vi "LevyLab Instrument.Configuration Window.vi"(8 "error in (no error)":errorcluster, 11 "Example Instrument in":refnum<class "Example.lvclass">) -> (0 "error out":errorcluster, 3 "Example Instrument out":refnum<class "Example.lvclass">)   [LabVIEW 2019, in "Example.lvclass"]
uses:
  Example.lvclass
  Example.lvclass/Example.ctl
panel:
  in  "Example Setting 3":string
  in  "Example Setting 2":dbl
  in  "Example Setting 1":dbl
  in  "Cancel":bool
  in  "OK":bool
  # "confirm or make changes:"
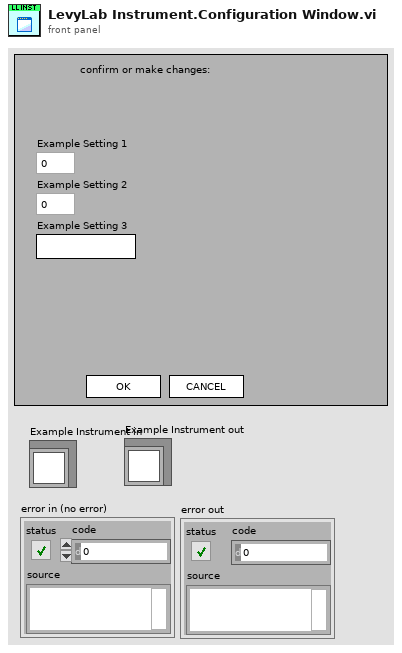
[diagram p1: front panel]
types:
  T1 = enum32{"Invalid", "Standard", "Closed", "Hidden", "Minimized", "Maximized"}
  T2 = enum32{"invalid app kind", "Development System", "Run Time System", "Student Edition", "Embedded LabVIEW", "Evaluation", "Custom"}
  T3 = typedef "Example.lvclass/LevyLab Instrument.Configuration--Cluster.ctl" = cluster{"Example Setting 1":dbl, "Example Setting 2":dbl, "Example Setting 3":string}
  T4 = cluster{"Core":cluster{"Current VI Reference":refnum<vi>, "Close Panel on Exit?":bool}, "Configuration":T3}
  T5 = cluster{"Current VI Reference":refnum<vi>, "Close Panel on Exit?":bool}
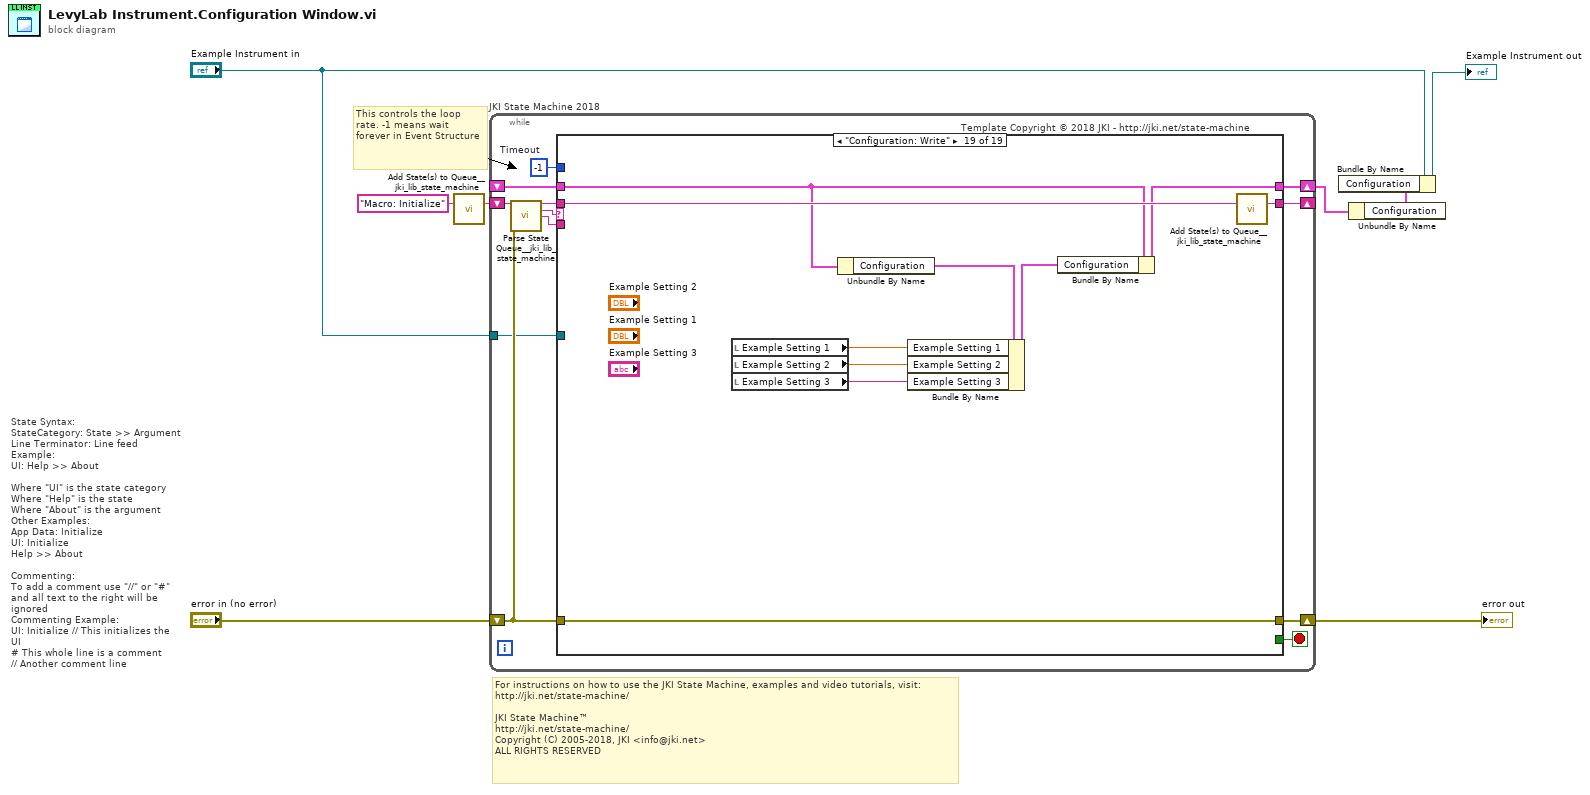
[diagram p0: block diagram]
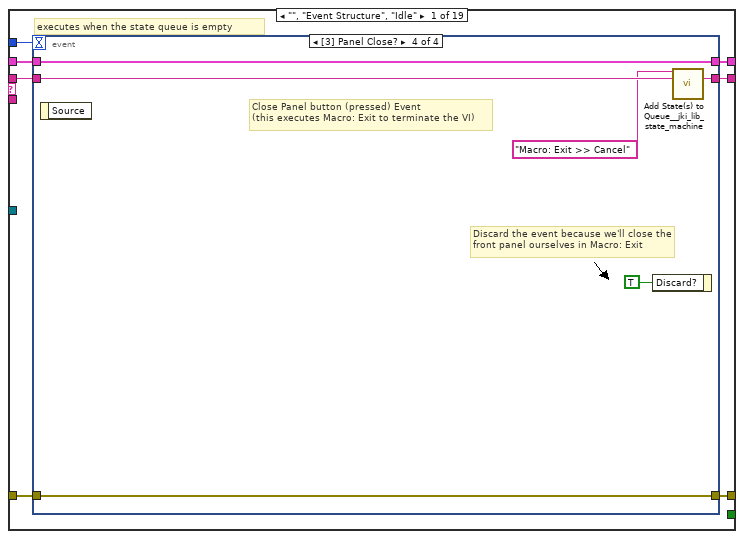
[diagram p2: hidden frame]
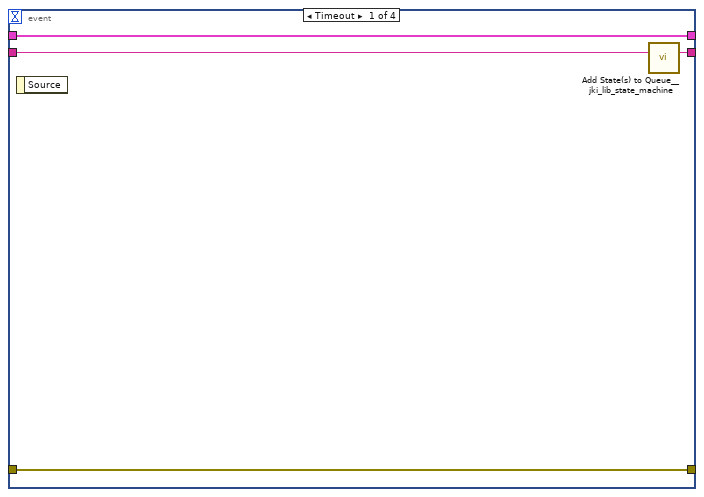
[diagram p3: hidden frame]
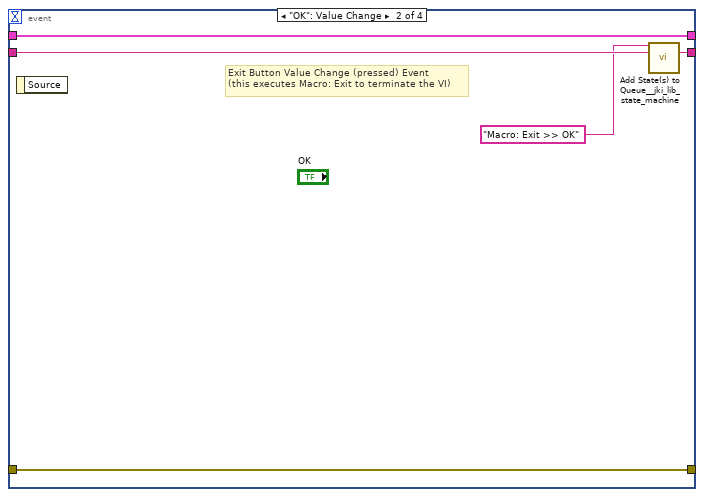
[diagram p4: hidden frame]
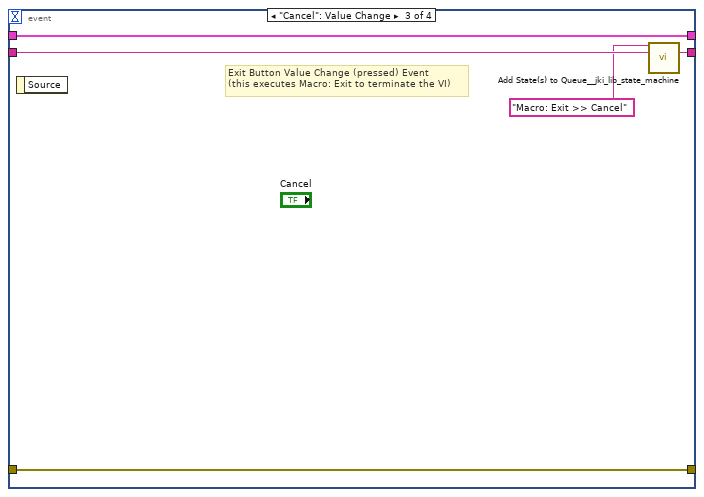
[diagram p5: hidden frame]
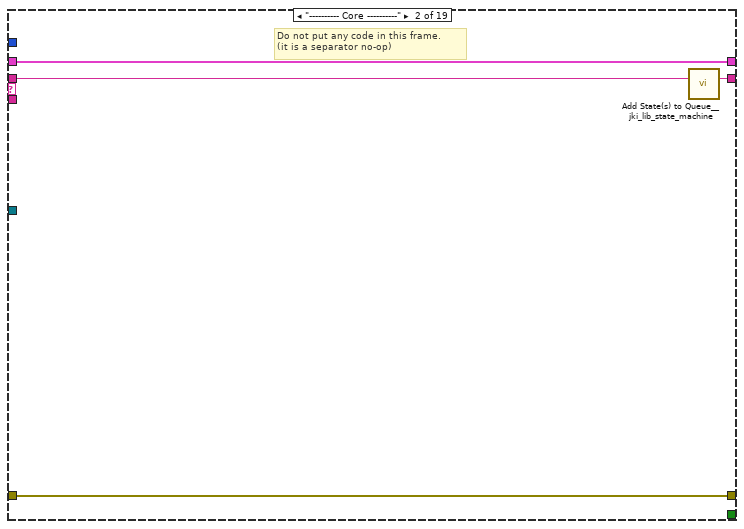
[diagram p6: hidden frame]
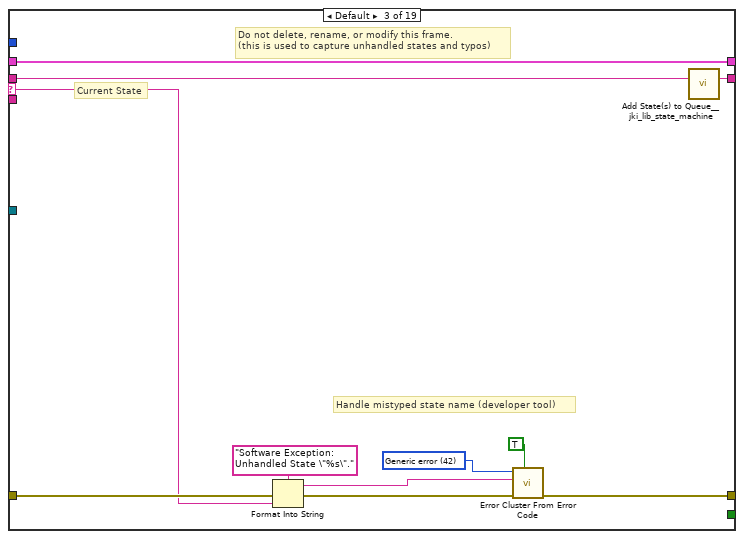
[diagram p7: hidden frame]
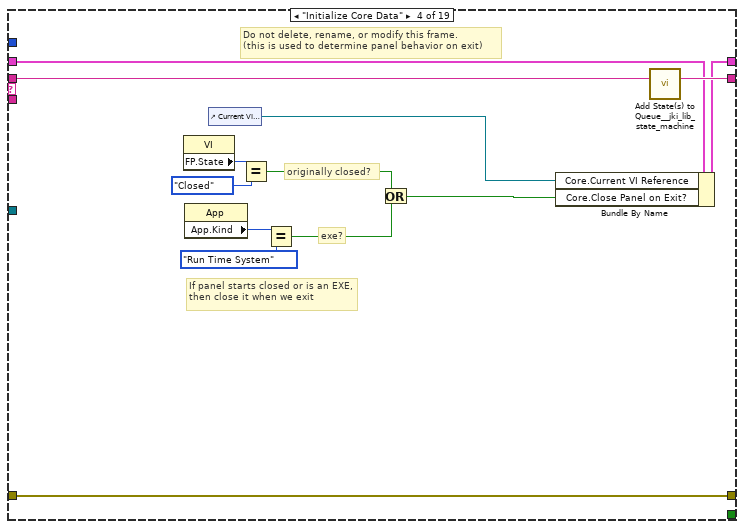
[diagram p8: hidden frame]
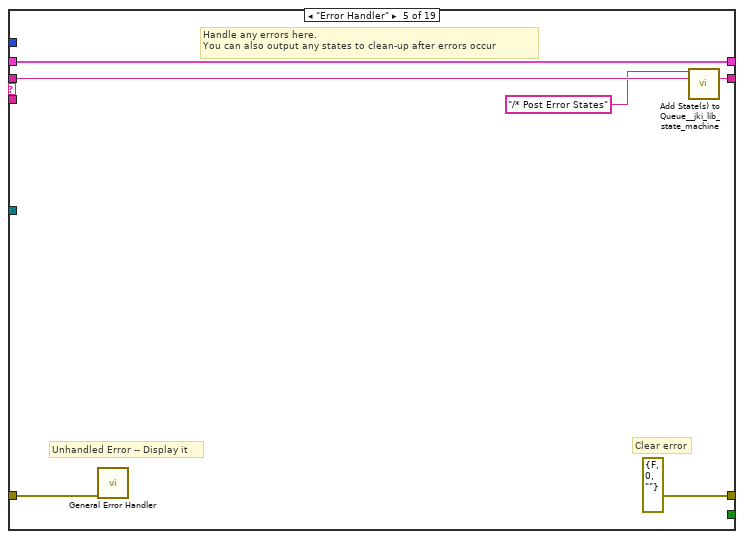
[diagram p9: hidden frame]
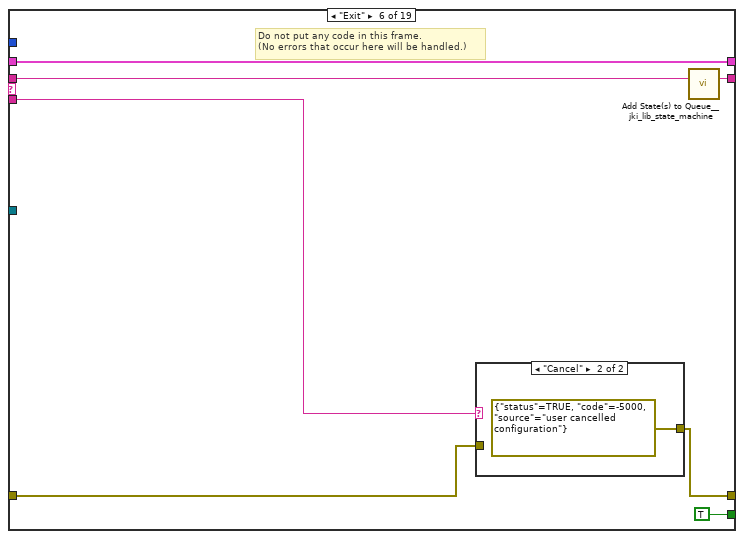
[diagram p10: hidden frame]
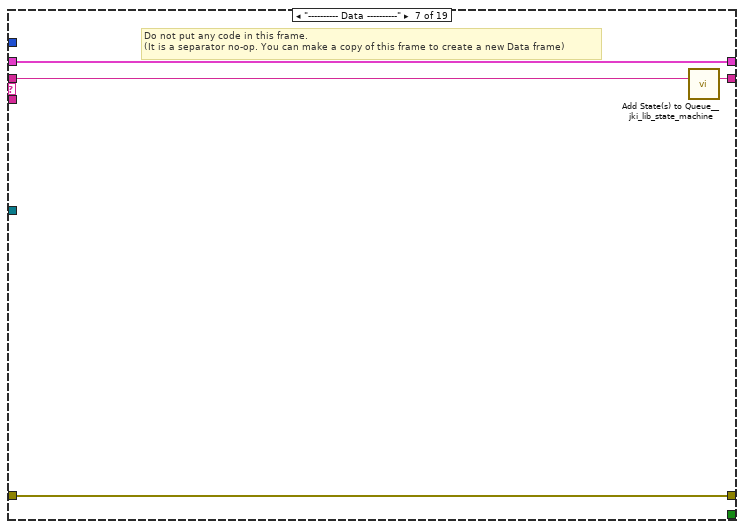
[diagram p12: hidden frame]
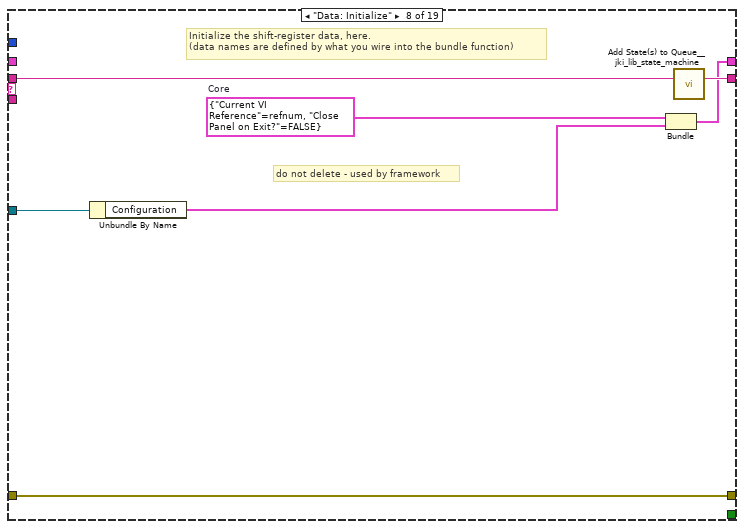
[diagram p13: hidden frame]
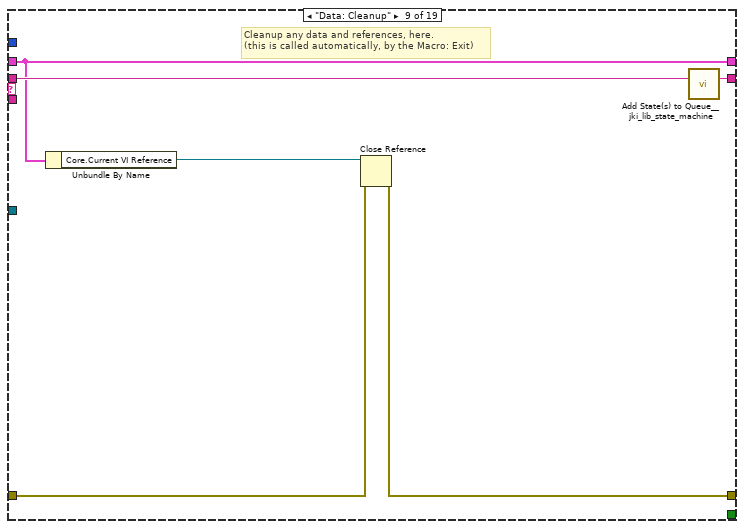
[diagram p14: hidden frame]
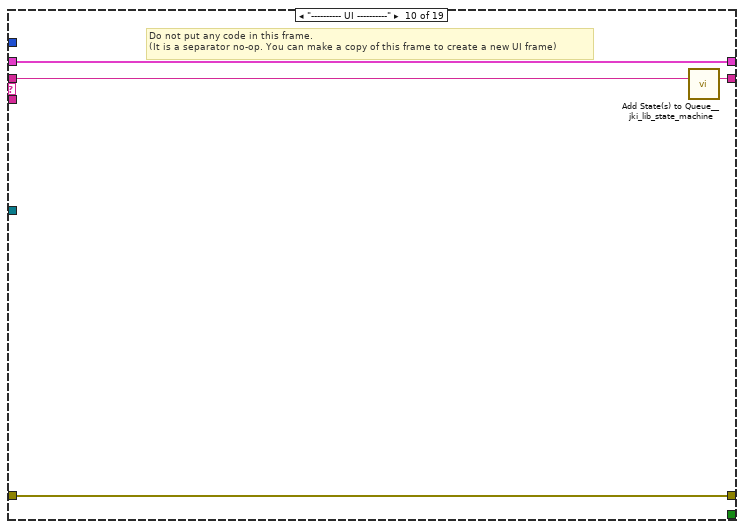
[diagram p15: hidden frame]
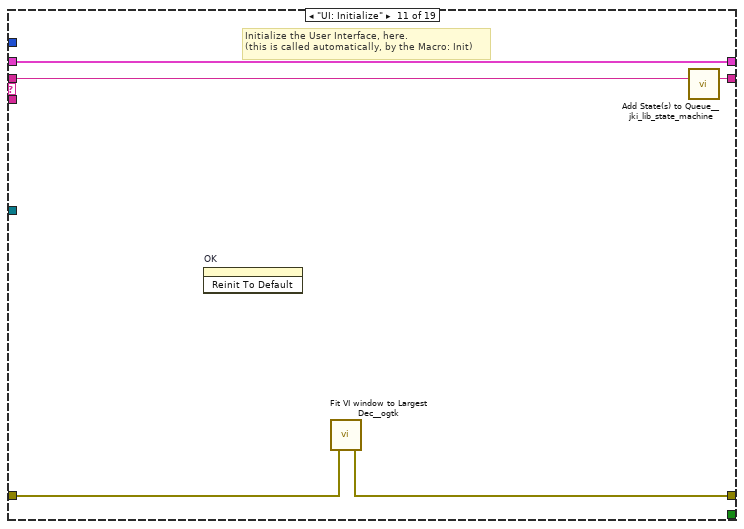
[diagram p16: hidden frame]
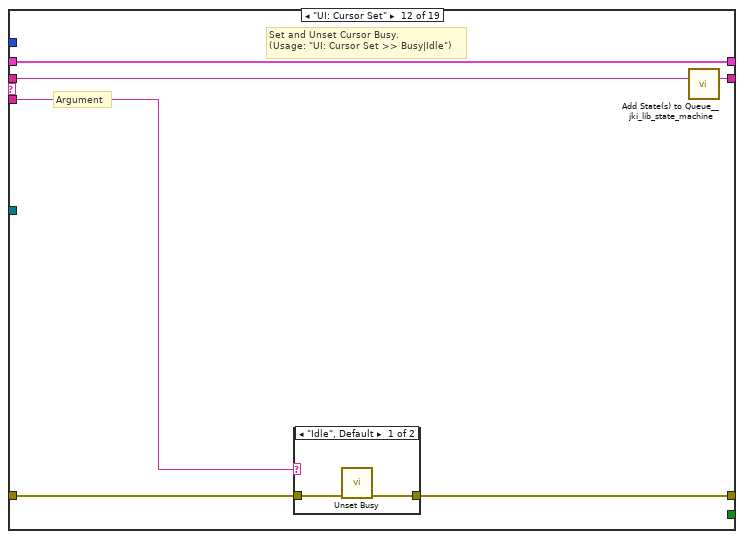
[diagram p17: hidden frame]
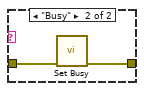
[diagram p18: hidden frame]
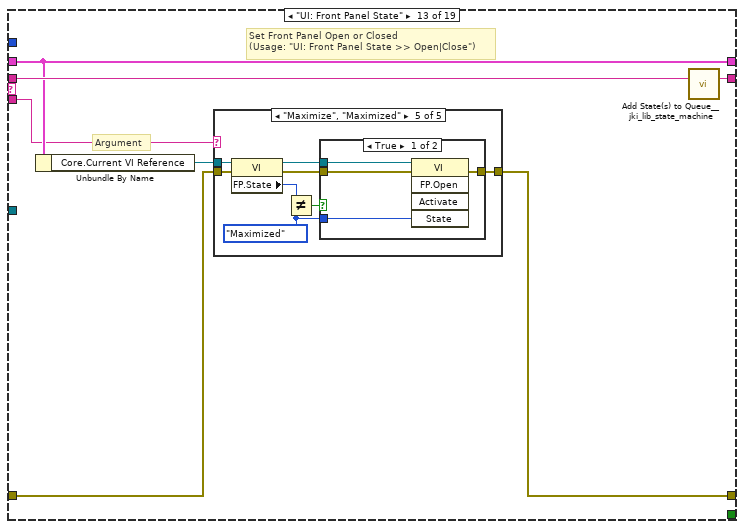
[diagram p19: hidden frame]
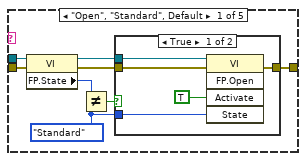
[diagram p20: hidden frame]
diagram:
  # "For instructions on how to use the JKI State Machine, examples and video tutorials, visit:\nhttp://jki.net/state-machine/\n\nJKI State Machine™\nhttp://jki.net/state-machine/\nCopyright (C) 2005-2018, JKI <info@jki.net>\nALL RIGHTS RESERVED"
  # "State Syntax:\nStateCategory: State >> Argument\nLine Terminator: Line feed\nExample:\nUI: Help >> About\n\nWhere \"UI\" is the state category\nWhere \"Help\" is the state\nWhere \"About\" is the argument\nOther Examples:\nApp Data: Initialize\nUI: Initialize\nHelp >> About\n\nCommenting:\nTo add a comment use \"//\" or \"#\" and all text to the right will be ignored\nCommenting Example:\nUI: Initialize // This initializes the UI\n# This whole line is a comment\n// Another comment line"
  # "This controls the loop rate. -1 means wait forever in Event Structure"
  n1 = call <vilib>:"Add State(s) to Queue__jki_lib_state_machine.vi"("State(s) in (\"\")"="Macro: Initialize") -> ("States Out"=w8:string)  [unwired: 14 in]
  n2 = while "JKI State Machine 2018" {
    shift-right: [w13] -> w2
    shift-left: _ -> [w12]
    shift-right: [w16] -> w6
    shift-left: "error in (no error)" -> [w10]
    shift-right: [w15] -> _
    shift-left: w8 -> [w17]
    tunnel: "Example Instrument in" -> [w9]
    stop <- w14 stop-if-true
    w11 = -1  # Timeout
    # "Template Copyright © 2018 JKI - http://jki.net/state-machine"
    n3 = call <vilib>:"Parse State Queue__jki_lib_state_machine.vi"("State Queue"=w17, "Error In (no error)"=w10) -> ("Remaining States"=w19:string, "Current State"=w20:string, "Arguments"=w18:string)  [unwired: 11 in]
    n4 = case shown="\"Configuration: Write\"" w20 {
      selector: w20 -> [_ _ w52 _ _ _ _ _ _ _ _ _ _ _ _ _ _ _ _]
      tunnel: w19 -> [w27 w51 w56 w75 w81 w88 w94 w101 w107 w111 w116 w122 w133 w202 w207 w222 w226 w234 w244]
      tunnel: w18 -> [_ _ _ _ _ w84 _ _ _ _ _ w117 w127 _ _ w211 _ _ _]
      tunnel: w12 -> [w25 w48 w54 w68 w78 w86 w91 _ w102 w108 w114 w120 w129 w199 w204 w219 w223 w228 w236]
      tunnel: [w24 w49 w58 w72 errorcluster {"status"=FALSE, "code"=0, "source"=""} ("error out") w82 w92 w97 w103 w109 w112 w118 w130 w200 w205 w220 w224 w232 w242] -> w16
      tunnel: w10 -> [w23 w49 w57 w72 w77 w83 w92 w97 w104 w109 w113 w119 w131 w200 w205 w220 w224 w232 w242]
      tunnel: [w26 w50 w55 w74 w80 w87 w93 w100 w106 w110 w115 w121 w132 w201 w206 w221 w225 w233 w243] -> w15
      tunnel: [_ _ _ _ _ TRUE _ _ _ _ _ _ _ _ _ _ _ _ _] -> w14
      tunnel: [w22 w48 w54 w73 w78 w86 w91 w99 w102 w108 w114 w120 w129 w199 w204 w219 w223 w228 w235] -> w13
      tunnel: w11 -> [w21 _ _ _ _ _ _ _ _ _ _ _ _ _ _ _ _ _ _]
      tunnel: w9 -> [_ _ _ _ _ _ _ w96 _ _ _ _ _ _ _ _ _ _ _]
      frame "", "Event Structure", "Idle" {
        # "executes when the state queue is empty"
        n5 = event shown="[3] Panel Close?" {
          selector: _ -> [_ _ _ _]
          dyn-events: _ -> [_ _ _ _]
          timeout: w21 -> [_ _ _ _]
          tunnel: w27 -> [w31 w36 w41 w47]
          tunnel: [w30 w35 w40 w46] -> w26
          tunnel: w25 -> [w28 w33 w38 w44]
          tunnel: [w29 w34 w39 w45] -> w24
          tunnel: w23 -> [w29 w34 w39 w45]
          tunnel: [w28 w33 w38 w44] -> w22
          event Timeout {
            n6 = event-data() -> ()  [unwired: 1 in, 1 out]
            n7 = call <vilib>:"Add State(s) to Queue__jki_lib_state_machine.vi"("State(s) in (\"\")"=w31) -> ("States Out"=w30:string)  [unwired: 14 in]
          }
          event "OK": Value Change {
            # "Exit Button Value Change (pressed) Event\n(this executes Macro: Exit to terminate the VI)"
            n8 = event-data() -> ()  [unwired: 1 in, 1 out]
            n9 = call <vilib>:"Add State(s) to Queue__jki_lib_state_machine.vi"("State(s) in Front (\"\")"="Macro: Exit >> OK", "State(s) in (\"\")"=w36) -> ("States Out"=w35:string)  [unwired: 13 in]
          }
          event "Cancel": Value Change {
            # "Exit Button Value Change (pressed) Event\n(this executes Macro: Exit to terminate the VI)"
            n10 = event-data() -> ()  [unwired: 1 in, 1 out]
            n11 = call <vilib>:"Add State(s) to Queue__jki_lib_state_machine.vi"("State(s) in Front (\"\")"="Macro: Exit >> Cancel", "State(s) in (\"\")"=w41) -> ("States Out"=w40:string)  [unwired: 13 in]
          }
          event Panel Close? {
            # "Discard the event because we'll close the front panel ourselves in Macro: Exit"
            # "Close Panel button (pressed) Event\n(this executes Macro: Exit to terminate the VI)"
            n12 = event-data() -> ()  [unwired: 1 in, 1 out]
            n13 = event-data("Discard?"=TRUE) -> ()  [unwired: 1 in, 1 out]
            n14 = call <vilib>:"Add State(s) to Queue__jki_lib_state_machine.vi"("State(s) in Front (\"\")"="Macro: Exit >> Cancel", "State(s) in (\"\")"=w47) -> ("States Out"=w46:string)  [unwired: 13 in]
          }
        }
      }
      frame "---------- Core ----------" {
        # "Do not put any code in this frame.\n(it is a separator no-op)"
        n15 = call <vilib>:"Add State(s) to Queue__jki_lib_state_machine.vi"("State(s) in (\"\")"=w51) -> ("States Out"=w50:string)  [unwired: 14 in]
      }
      frame Default {
        w61 = 42 items=["No error", "Argument error", "Memory is full", "Out of zone", "End of file", "File already open", "Generic file I/O error", "File not found", "File permission error", "Disk is full", "Duplicate path", "Too many files open", "System feature not enabled", "Resource file not found", "Cannot add resource", "Resource not found", "Image not found", "Image memory error", "Pen does not exist", "Config type invalid", "Config token not found", "Config parse error", "Config memory error", "Bad external code format", "Bad external code offset", "External code not present", "Null window", "Destroy window error", "Null menu", "Print aborted", "Bad print record", "Print driver error", "Windows error during printing", "Memory error during printing", "Print dialog error", "Generic print error", "Invalid device refnum", "Device not found", "Device parameter error", "Device unit error", "Cannot open device", "Device call aborted", "Generic error", "Cancelled by user", "Object ID too low", "Object ID too high", "Object not in heap", "Unknown heap", "Unknown object (invalid DefProc)", "Unknown object (DefProc not in table)", "Message out of range", "Invalid (null) method", "Unknown message", "Manager call not supported", "Bad address", "Network operation in progress", "Network operation timed out", "Connection is busy", "Network attribute not supported", "Network error", "Address in use", "System out of memory", "Connection aborted", "Connection refused", "Not connected", "Already connected", "Connection closed", "Initialization error (interapplication manager)", "Bad occurrence", "Wait on unbound occurrence handler", "Occurrence queue overflow", "Datalog type conflict", "Unused", "Unrecognized type (interapplication manager)", "Memory corrupt", "Failed to make temporary DLL", "Old CIN version", "Drag socket not found", "Failed to load drop-object", "Failed to register OLE object", "Failed to release OLE object", "Format specifier type mismatch", "Unknown format specifier", "Too few format specifiers", "Too many format specifiers", "Scan failed", "Newer CIN version", "Error converting to variant", "Runtime menu error", "Password tampered", "Variant attribute not found", "Incompatible variant data type", "Event data is not available", "Event Store is not present", "Occurrence is not found", "Event Queue is not created", "Event info is not available", "Refnum passed is NULL", "Error retrieving Class GUID", "Error retrieving CoClass GUID", "Error retrieving TypeLib GUID.", "Bad built application magic bytes.", "Specific driver is different from the specific driver associated with the Logical Name.", "There is no session opened to the class driver.", "Max Error", "MAX - Error with config objects", "MAX - Error loading configuration", "MAX - Group not supported"]
        # "Current State"
        # "Do not delete, rename, or modify this frame.\n(this is used to capture unhandled states and typos)"
        # "Handle mistyped state name (developer tool)"
        n16 = Format Into String(format string="Software Exception: Unhandled State \"%s\"." ("message"), error in=w57, w52) -> (resulting string=w60:string, error out=w59:errorcluster)  [unwired: 1 in]
        n17 = call <vilib>:"Error Cluster From Error Code.vi"("show call chain? (False)"=TRUE, "error in (no error)"=w59, "error message (\"\")"=w60, "error code (0)"=w61) -> ("error out"=w58:errorcluster)  [unwired: 5 in]
        n18 = call <vilib>:"Add State(s) to Queue__jki_lib_state_machine.vi"("State(s) in (\"\")"=w56) -> ("States Out"=w55:string)  [unwired: 14 in]
      }
      frame "Initialize Core Data" {
        # "Do not delete, rename, or modify this frame.\n(this is used to determine panel behavior on exit)"
        # "originally closed?"
        # "exe?"
        # "If panel starts closed or is an EXE, then close it when we exit"
        n19 = property class="VI"() -> ("FP.State"=w65:T1)  [unwired: 2 in, 2 out]
        n20 = property class="App"() -> ("App.Kind"=w71:T2)  [unwired: 2 in, 2 out]
        n21 = control-ref of="Current VI Reference"() -> (w66:refnum<vi>)
        n22 = Equal?(x=w65, y=T1."Closed" ("Front Panel Window:State")) -> (x = y?=w63:bool)
        n23 = Equal?(x=w71, y=T2."Run Time System" ("Application:Kind")) -> (x = y?=w69:bool)
        n24 = Or(x=w63, y=w69) -> (x .or. y?=w67:bool)
        n25 = Bundle By Name(cluster=w68, "Core.Current VI Reference"=w66, "Core.Close Panel on Exit?"=w67) -> (w73:T4)
        n26 = call <vilib>:"Add State(s) to Queue__jki_lib_state_machine.vi"("State(s) in (\"\")"=w75) -> ("States Out"=w74:string)  [unwired: 14 in]
      }
      frame "Error Handler" {
        # "Unhandled Error -- Display it"
        # "Handle any errors here.\nYou can also output any states to clean-up after errors occur"
        # "Clear error"
        n27 = call <vilib>:"General Error Handler.vi"("error in (no error)"=w77) -> ()  [unwired: 10 in, 5 out]
        n28 = call <vilib>:"Add State(s) to Queue__jki_lib_state_machine.vi"("State(s) in Front (\"\")"="/* Post Error States", "State(s) in (\"\")"=w81) -> ("States Out"=w80:string)  [unwired: 13 in]
      }
      frame "Exit" {
        # "Do not put any code in this frame.\n(No errors that occur here will be handled.)"
        n29 = case shown="\"Cancel\"" w84 {
          tunnel: w83 -> [w89 _]
          tunnel: [w89 errorcluster {"status"=TRUE, "code"=-5000, "source"="user cancelled configuration"} ("error in (no error)")] -> w82
          frame "OK", Default {
          }
          frame "Cancel" {
          }
        }
        n30 = call <vilib>:"Add State(s) to Queue__jki_lib_state_machine.vi"("State(s) in (\"\")"=w88) -> ("States Out"=w87:string)  [unwired: 14 in]
      }
      frame "---------- Data ----------" {
        # "Do not put any code in this frame.\n(It is a separator no-op. You can make a copy of this frame to create a new Data frame)"
        n31 = call <vilib>:"Add State(s) to Queue__jki_lib_state_machine.vi"("State(s) in (\"\")"=w94) -> ("States Out"=w93:string)  [unwired: 14 in]
      }
      frame "Data: Initialize" {
        w98 = T5 {"Current VI Reference"=refnum, "Close Panel on Exit?"=FALSE}  # Core
        # "do not delete - used by framework"
        # "Initialize the shift-register data, here.\n(data names are defined by what you wire into the bundle function)"
        n32 = Unbundle By Name(w96) -> ("Configuration"=w95:T3)
        n33 = Bundle("Core"=w98, "Configuration"=w95) -> (w99:T4)  [unwired: 1 in]
        n34 = call <vilib>:"Add State(s) to Queue__jki_lib_state_machine.vi"("State(s) in (\"\")"=w101) -> ("States Out"=w100:string)  [unwired: 14 in]
      }
      frame "Data: Cleanup" {
        # "Cleanup any data and references, here.\n(this is called automatically, by the Macro: Exit)"
        n35 = Unbundle By Name(w102) -> ("Core.Current VI Reference"=w105:refnum<vi>)
        n36 = Close Reference(reference=w105, error in (no error)=w104) -> (error out=w103:errorcluster)
        n37 = call <vilib>:"Add State(s) to Queue__jki_lib_state_machine.vi"("State(s) in (\"\")"=w107) -> ("States Out"=w106:string)  [unwired: 14 in]
      }
      frame "---------- UI ----------" {
        # "Do not put any code in this frame.\n(It is a separator no-op. You can make a copy of this frame to create a new UI frame)"
        n38 = call <vilib>:"Add State(s) to Queue__jki_lib_state_machine.vi"("State(s) in (\"\")"=w111) -> ("States Out"=w110:string)  [unwired: 14 in]
      }
      frame "UI: Initialize" {
        # "Initialize the User Interface, here.\n(this is called automatically, by the Macro: Init)"
        n39 = invoke on="OK" class="Bool" method="Reinit To Default"() -> ()  [unwired: 3 in, 3 out]
        n40 = call <userlib>:"Fit VI window to Largest Dec__ogtk.vi"("error in (no error)"=w113) -> ("error out"=w112:errorcluster)  [unwired: 5 in, 1 out]
        n41 = call <vilib>:"Add State(s) to Queue__jki_lib_state_machine.vi"("State(s) in (\"\")"=w116) -> ("States Out"=w115:string)  [unwired: 14 in]
      }
      frame "UI: Cursor Set" {
        # "Argument"
        # "Set and Unset Cursor Busy.\n(Usage: \"UI: Cursor Set >> Busy|Idle\")"
        n42 = case shown="\"Idle\", Default" w117 {
          tunnel: w119 -> [w124 w126]
          tunnel: [w123 w125] -> w118
          frame "Idle", Default {
            n43 = call <vilib>:"Unset Busy.vi"("error in (no error)"=w124) -> ("error out"=w123:errorcluster)  [unwired: 10 in]
          }
          frame "Busy" {
            n44 = call <vilib>:"Set Busy.vi"("error in (no error)"=w126) -> ("error out"=w125:errorcluster)  [unwired: 9 in, 1 out]
          }
        }
        n45 = call <vilib>:"Add State(s) to Queue__jki_lib_state_machine.vi"("State(s) in (\"\")"=w122) -> ("States Out"=w121:string)  [unwired: 14 in]
      }
      frame "UI: Front Panel State" {
        # "Argument"
        # "Set Front Panel Open or Closed\n(Usage: \"UI: Front Panel State >> Open|Close\")"
        n46 = Unbundle By Name(w129) -> ("Core.Current VI Reference"=w128:refnum<vi>)
        n47 = case shown="\"Maximize\", \"Maximized\"" w127 {
          tunnel: w131 -> [w139 w154 w165 w178 w191]
          tunnel: [w141 w155 w167 w180 w193] -> w130
          tunnel: w128 -> [w140 w152 w166 w179 w192]
          frame "Open", "Standard", Default {
            w134 = T1."Standard" ("State")
            n48 = property class="VI"(reference=w140, error in=w139) -> (reference out=w137:refnum<vi>, error out=w138:errorcluster, "FP.State"=w136:T1)
            n49 = Not Equal?(x=w136, y=w134) -> (x != y?=w135:bool)
            n50 = case shown="True" w135 {
              tunnel: [w145 w147] -> w141
              tunnel: w138 -> [w144 w147]
              tunnel: w137 -> [w143 _]
              tunnel: w134 -> [w142 _]
              frame True {
                n51 = invoke class="VI" method="FP.Open"(reference=w143, error in=w144, "Activate"=TRUE, "State"=w142) -> (error out=w145:errorcluster)  [unwired: 1 in, 4 out]
              }
              frame False {
              }
            }
          }
          frame "Close", "Closed" {
            n52 = property class="VI"(reference=w152, error in=w154) -> (reference out=w151:refnum<vi>, error out=w153:errorcluster, "FP.State"=w149:T1)
            n53 = Not Equal?(x=w149, y=T1."Closed" ("Front Panel Window:State")) -> (x != y?=w148:bool)
            n54 = case shown="True" w148 {
              tunnel: [w156 w159] -> w155
              tunnel: w153 -> [w156 w158]
              tunnel: w151 -> [_ w157]
              frame False {
              }
              frame True {
                n55 = invoke class="VI" method="FP.Close"(reference=w157, error in=w158) -> (error out=w159:errorcluster)  [unwired: 1 in, 2 out]
              }
            }
          }
          frame "Hidden", "Hide" {
            w160 = T1."Hidden" ("State")
            n56 = property class="VI"(reference=w166, error in=w165) -> (reference out=w163:refnum<vi>, error out=w164:errorcluster, "FP.State"=w162:T1)
            n57 = Not Equal?(x=w162, y=w160) -> (x != y?=w161:bool)
            n58 = case shown="True" w161 {
              tunnel: [w171 w172] -> w167
              tunnel: w164 -> [w170 w172]
              tunnel: w163 -> [w169 _]
              tunnel: w160 -> [w168 _]
              frame True {
                n59 = invoke class="VI" method="FP.Open"(reference=w169, error in=w170, "State"=w168) -> (error out=w171:errorcluster)  [unwired: 2 in, 4 out]
              }
              frame False {
              }
            }
          }
          frame "Minimize", "Minimized" {
            w173 = T1."Minimized" ("State")
            n60 = property class="VI"(reference=w179, error in=w178) -> (reference out=w176:refnum<vi>, error out=w177:errorcluster, "FP.State"=w175:T1)
            n61 = Not Equal?(x=w175, y=w173) -> (x != y?=w174:bool)
            n62 = case shown="True" w174 {
              tunnel: [w184 w185] -> w180
              tunnel: w177 -> [w183 w185]
              tunnel: w176 -> [w182 _]
              tunnel: w173 -> [w181 _]
              frame True {
                n63 = invoke class="VI" method="FP.Open"(reference=w182, error in=w183, "State"=w181) -> (error out=w184:errorcluster)  [unwired: 2 in, 4 out]
              }
              frame False {
              }
            }
          }
          frame "Maximize", "Maximized" {
            w186 = T1."Maximized" ("State")
            n64 = property class="VI"(reference=w192, error in=w191) -> (reference out=w189:refnum<vi>, error out=w190:errorcluster, "FP.State"=w188:T1)
            n65 = Not Equal?(x=w188, y=w186) -> (x != y?=w187:bool)
            n66 = case shown="True" w187 {
              tunnel: [w197 w198] -> w193
              tunnel: w190 -> [w196 w198]
              tunnel: w189 -> [w195 _]
              tunnel: w186 -> [w194 _]
              frame True {
                n67 = invoke class="VI" method="FP.Open"(reference=w195, error in=w196, "State"=w194) -> (error out=w197:errorcluster)  [unwired: 2 in, 4 out]
              }
              frame False {
              }
            }
          }
        }
        n68 = call <vilib>:"Add State(s) to Queue__jki_lib_state_machine.vi"("State(s) in (\"\")"=w133) -> ("States Out"=w132:string)  [unwired: 14 in]
      }
      frame "---------- Macro ----------" {
        # "Do not put any code in this frame.\n(It is a separator no-op. You can make a copy of this frame to create a new Macro frame)"
        n69 = call <vilib>:"Add State(s) to Queue__jki_lib_state_machine.vi"("State(s) in (\"\")"=w202) -> ("States Out"=w201:string)  [unwired: 14 in]
      }
      frame "Macro: Initialize" {
        w203 = "Data: Initialize\nInitialize Core Data\nUI: Initialize\nUI: Front Panel State >> Open\nConfiguration: Read"  # Data: Initialize Initialize Core Data UI: Initialize UI: Front Panel State >> Open Configuration: Read
        # "Initialization Macro\n(This is called once, when the VI starts)"
        n70 = call <vilib>:"Add State(s) to Queue__jki_lib_state_machine.vi"("State(s) in Front (\"\")"=w203, "State(s) in (\"\")"=w207) -> ("States Out"=w206:string)  [unwired: 13 in]
      }
      frame "Macro: Exit" {
        # "Exit Macro\n(This is called once, when the VI exits)"
        n71 = Unbundle By Name(w219) -> ("Core.Close Panel on Exit?"=w218:bool)
        n72 = call <vilib>:"Build State String with Arguments__JKI_lib_State_Machine.vi"("Arguments (\"\")"=w211, "State"="Exit") -> ("State with Arguments"=w209:string)  [unwired: 4 in]
        n73 = Select(t="UI: Front Panel State >> Close", s=w218, f="") -> (s? t:f=w215:string)
        n74 = call <vilib>:"Add State(s) to Queue__jki_lib_state_machine.vi"("State(s) in Front (\"\")"="Data: Cleanup", "State(s) at Back (\"\")"=w209) -> ("States Out"=w208:string)  [unwired: 13 in]
        n75 = call <vilib>:"Add State(s) to Queue__jki_lib_state_machine.vi"("State(s) in Front (\"\")"="Configuration: Write", "State(s) in (\"\")"=w215, "State(s) at Back (\"\")"=w208) -> ("States Out"=w214:string)  [unwired: 12 in]
        n76 = call <vilib>:"Add State(s) to Queue__jki_lib_state_machine.vi"("State(s) in Front (\"\")"=w214, "State(s) in (\"\")"=w222) -> ("States Out"=w221:string)  [unwired: 13 in]
      }
      frame "---------- Configuration ----------" {
        # "Template Separator\n(You can make a copy of, or modify, this frame)"
        n77 = call <vilib>:"Add State(s) to Queue__jki_lib_state_machine.vi"("State(s) in (\"\")"=w226) -> ("States Out"=w225:string)  [unwired: 14 in]
      }
      frame "Configuration: Read" {
        # "Your code here.\n(You can make a copy of, or modify, this frame)"
        n78 = Unbundle By Name(w228) -> ("Configuration"=w227:T3)
        n79 = Unbundle By Name(w227) -> ("Example Setting 1"=w231:dbl, "Example Setting 2"=w230:dbl, "Example Setting 3"=w229:string)
        n80 = local write "Example Setting 2"(w230) -> ()
        n81 = local write "Example Setting 1"(w231) -> ()
        n82 = local write "Example Setting 3"(w229) -> ()
        n83 = call <vilib>:"Add State(s) to Queue__jki_lib_state_machine.vi"("State(s) in (\"\")"=w234) -> ("States Out"=w233:string)  [unwired: 14 in]
      }
      frame "Configuration: Write" {
        n84 = local read "Example Setting 1"() -> (w241:dbl)
        n85 = local read "Example Setting 2"() -> (w238:dbl)
        n86 = local read "Example Setting 3"() -> (w239:string)
        n87 = Unbundle By Name(w236) -> ("Configuration"=w240:T3)
        n88 = Bundle By Name(cluster=w240, "Example Setting 1"=w241, "Example Setting 2"=w238, "Example Setting 3"=w239) -> (w237:T3)
        n89 = Bundle By Name(cluster=w236, "Configuration"=w237) -> (w235:T4)
        n90 = call <vilib>:"Add State(s) to Queue__jki_lib_state_machine.vi"("State(s) in (\"\")"=w244) -> ("States Out"=w243:string)  [unwired: 14 in]
      }
    }
  }
  "error out" <- w6
  n91 = Unbundle By Name(w2) -> ("Configuration"=w1:T3)
  n92 = Bundle By Name(cluster="Example Instrument in", "Configuration"=w1) -> (→"Example Instrument out":refnum<class "Example.lvclass">)
